vi "try3.vi"() -> ()   [LabVIEW 2023]
panel:
  in  "file path (use dialog)":path
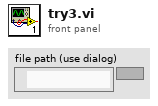
[diagram p1: front panel]
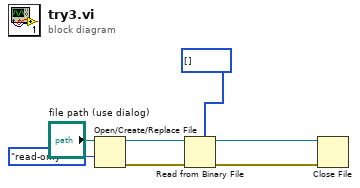
[diagram p0: block diagram]
diagram:
  n1 = Open/Create/Replace File(file path (use dialog)="file path (use dialog)", access (0:read/write)=enum16{"read/write", "read-only", "write-only"}."read-only") -> (refnum out=w6:refnum<file>, error out=w5:errorcluster)  [unwired: 4 in, 1 out]
  n2 = Read from Binary File(5:i8[] [], 8:w5, 11:w6) -> (0:w3:errorcluster, 3:w4:refnum<file>)  [unwired: 3 in, 2 out]
  n3 = Close File(refnum=w4, error in=w3) -> ()  [unwired: 2 out]
